vi "Save Project.vi"(0 "Project reference":refnum<vi>, 5 "MeasurementCore reference":refnum<vi>, 7 "Project path":path, 11 "error in (no error)":errorcluster) -> (15 "error out":errorcluster)   [LabVIEW 2021, in "Multiple Converter.lvlib"]
uses:
  Multiple Converter.lvlib
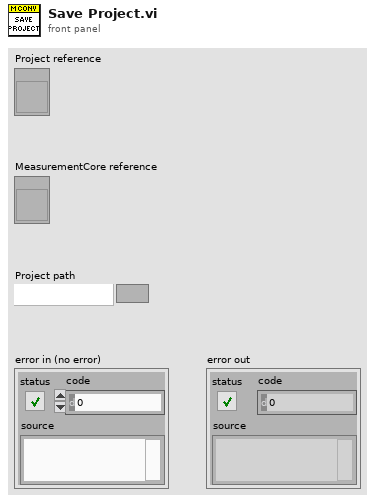
[diagram p1: front panel]
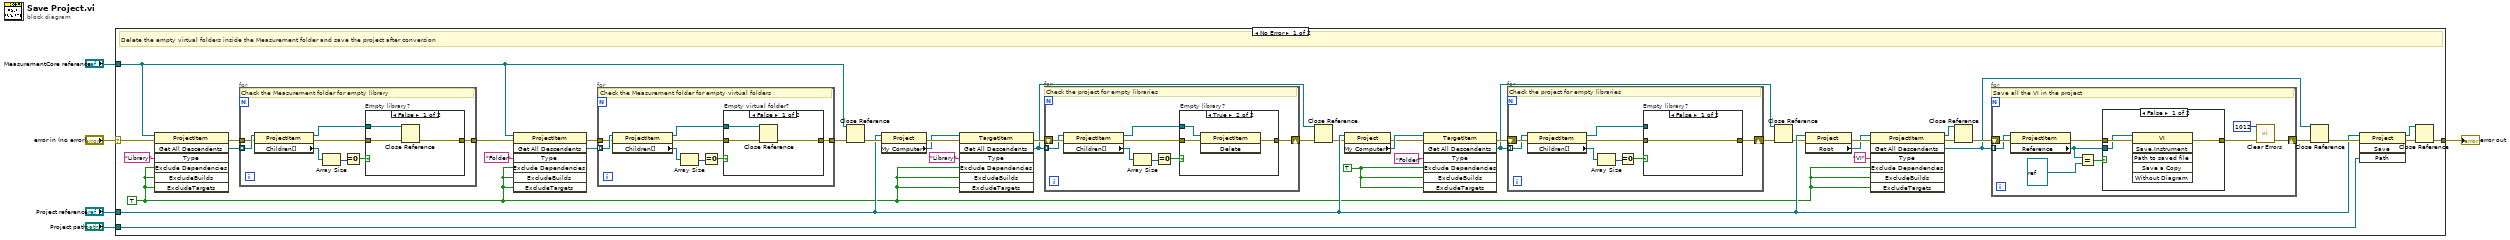
[diagram p0: block diagram]
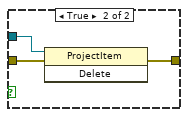
[diagram p2: hidden frame]
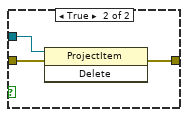
[diagram p3: hidden frame]
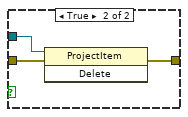
[diagram p4: hidden frame]
diagram:
  n1 = case shown="No Error" "error in (no error)" {
    selector: "error in (no error)" -> [w9 w112]
    tunnel: [w45 w112] -> w5
    tunnel: "Project path" -> [w41 _]
    tunnel: "MeasurementCore reference" -> [w6 _]
    tunnel: "Project reference" -> [w19 _]
    frame No Error {
      w7 = TRUE
      w18 = TRUE
      # "Delete the empty virtual folders inside the Measurement folder and save the project after conversion"
      n2 = invoke class="ProjectItem" method="Get All Descendents"(reference=w6, error in=w9, "Type"="Library", "Exclude Dependencies"=w7, "ExcludeBuilds"=w7, "ExcludeTargets"=w7) -> (error out=w11:errorcluster, "All Descendents"=w12:refnum<vi>[])  [unwired: 1 in, 5 out]
      n3 = for {
        tunnel: w12 -> [w54] mode=indexing
        tunnel: w11 -> [w53]
        tunnel: [w47] -> w8
        # "Check the Measurement folder for empty library"
        n4 = property class="ProjectItem"(reference=w54, error in=w53) -> (reference out=w48:refnum<vi>, error out=w50:errorcluster, "Children[]"=w52:refnum<vi>[])
        n5 = Array Size(array=w52) -> (size(s)=w51:i32)
        n6 = Equal To 0?(x=w51) -> (x = 0?=w49:bool)
        n7 = case "Empty library?" shown="False" w49 {
          tunnel: w50 -> [w57 w60]
          tunnel: w48 -> [w56 w59]
          tunnel: [w55 w58] -> w47
          frame False {
            n8 = Close Reference(reference=w56, error in (no error)=w57) -> (error out=w55:errorcluster)
          }
          frame True {
            n9 = invoke class="ProjectItem" method="Delete"(reference=w59, error in=w60) -> (error out=w58:errorcluster)  [unwired: 1 in, 2 out]
          }
        }
      }
      n10 = invoke class="ProjectItem" method="Get All Descendents"(reference=w6, error in=w8, "Type"="Folder", "Exclude Dependencies"=w7, "ExcludeBuilds"=w7, "ExcludeTargets"=w7) -> (error out=w42:errorcluster, "All Descendents"=w31:refnum<vi>[])  [unwired: 1 in, 5 out]
      n11 = for {
        tunnel: w31 -> [w80] mode=indexing
        tunnel: w42 -> [w79]
        tunnel: [w73] -> w24
        # "Check the Measurement folder for empty virtual folders"
        n12 = property class="ProjectItem"(reference=w80, error in=w79) -> (reference out=w74:refnum<vi>, error out=w76:errorcluster, "Children[]"=w78:refnum<vi>[])
        n13 = Array Size(array=w78) -> (size(s)=w77:i32)
        n14 = Equal To 0?(x=w77) -> (x = 0?=w75:bool)
        n15 = case "Empty virtual folder?" shown="False" w75 {
          tunnel: w76 -> [w83 w86]
          tunnel: w74 -> [w82 w85]
          tunnel: [w81 w84] -> w73
          frame False {
            n16 = Close Reference(reference=w82, error in (no error)=w83) -> (error out=w81:errorcluster)
          }
          frame True {
            n17 = invoke class="ProjectItem" method="Delete"(reference=w85, error in=w86) -> (error out=w84:errorcluster)  [unwired: 1 in, 2 out]
          }
        }
      }
      n18 = Close Reference(reference=w6, error in (no error)=w24) -> (error out=w23:errorcluster)
      n19 = property class="Project"(reference=w19, error in=w23) -> (error out=w35:errorcluster, "My Computer"=w25:refnum<vi>)  [unwired: 1 out]
      n20 = invoke class="TargetItem" method="Get All Descendents"(reference=w25, error in=w35, "Type"="Library", "Exclude Dependencies"=w7, "ExcludeBuilds"=w7, "ExcludeTargets"=w7) -> (error out=w33:errorcluster, "All Descendents"=w29:refnum<vi>[])  [unwired: 1 in, 5 out]
      n21 = for {
        shift-right: [w87] -> w30
        shift-left: w33 -> [w94]
        tunnel: w29 -> [w93] mode=indexing
        # "Check the project for empty libraries"
        n22 = property class="ProjectItem"(reference=w93, error in=w94) -> (reference out=w89:refnum<vi>, error out=w88:errorcluster, "Children[]"=w91:refnum<vi>[])
        n23 = Array Size(array=w91) -> (size(s)=w92:i32)
        n24 = Equal To 0?(x=w92) -> (x = 0?=w90:bool)
        n25 = case "Empty library?" shown="True" w90 {
          tunnel: w88 -> [w95 w98]
          tunnel: w89 -> [_ w97]
          tunnel: [w95 w96] -> w87
          frame False {
          }
          frame True {
            n26 = invoke class="ProjectItem" method="Delete"(reference=w97, error in=w98) -> (error out=w96:errorcluster)  [unwired: 1 in, 2 out]
          }
        }
      }
      n27 = Close Reference(reference=w29, error in (no error)=w30) -> (error out=w17:errorcluster)
      n28 = property class="Project"(reference=w19, error in=w17) -> (error out=w20:errorcluster, "My Computer"=w22:refnum<vi>)  [unwired: 1 out]
      n29 = invoke class="TargetItem" method="Get All Descendents"(reference=w22, error in=w20, "Type"="Folder", "Exclude Dependencies"=w18, "ExcludeBuilds"=w18, "ExcludeTargets"=w18) -> (error out=w16:errorcluster, "All Descendents"=w13:refnum<vi>[])  [unwired: 1 in, 5 out]
      n30 = for {
        shift-right: [w61] -> w15
        shift-left: w16 -> [w68]
        tunnel: w13 -> [w67] mode=indexing
        # "Check the project for empty libraries"
        n31 = property class="ProjectItem"(reference=w67, error in=w68) -> (reference out=w63:refnum<vi>, error out=w62:errorcluster, "Children[]"=w65:refnum<vi>[])
        n32 = Array Size(array=w65) -> (size(s)=w66:i32)
        n33 = Equal To 0?(x=w66) -> (x = 0?=w64:bool)
        n34 = case "Empty library?" shown="False" w64 {
          tunnel: w62 -> [w69 w72]
          tunnel: w63 -> [_ w71]
          tunnel: [w69 w70] -> w61
          frame False {
          }
          frame True {
            n35 = invoke class="ProjectItem" method="Delete"(reference=w71, error in=w72) -> (error out=w70:errorcluster)  [unwired: 1 in, 2 out]
          }
        }
      }
      n36 = Close Reference(reference=w13, error in (no error)=w15) -> (error out=w14:errorcluster)
      n37 = property class="Project"(reference=w19, error in=w14) -> (error out=w40:errorcluster, "Root"=w39:refnum<vi>)  [unwired: 1 out]
      n38 = invoke class="ProjectItem" method="Get All Descendents"(reference=w39, error in=w40, "Type"="VI", "Exclude Dependencies"=w7, "ExcludeBuilds"=w7, "ExcludeTargets"=w7) -> (reference out=w37:refnum<vi>, error out=w38:errorcluster, "All Descendents"=w26:refnum<vi>[])  [unwired: 1 in, 4 out]
      n39 = Close Reference(reference=w37, error in (no error)=w38) -> (error out=w36:errorcluster)
      n40 = for {
        shift-right: [w100] -> w28
        shift-left: w36 -> [w106]
        tunnel: w26 -> [w104] mode=indexing
        # "Save all the VI in the project"
        n41 = property class="ProjectItem"(reference=w104, error in=w106) -> (error out=w105:errorcluster, "Reference"=w101:refnum<vi>)  [unwired: 1 out]
        n42 = Equal?(x=w101, y=refnum<vi> refnum) -> (x = y?=w102:bool)
        n43 = case shown="False" w102 {
          tunnel: [w108 w111] -> w107
          tunnel: w105 -> [w110 w111]
          tunnel: w101 -> [w109 _]
          frame False {
            n44 = invoke class="VI" method="Save.Instrument"(reference=w109, error in=w110) -> (error out=w108:errorcluster)  [unwired: 4 in, 5 out]
          }
          frame True {
          }
        }
        n45 = call <vilib>:"Clear Errors.vi"("error in (no error)"=w107, "specific error code to clear (0: all)"=1012) -> ("error out"=w100:errorcluster)  [unwired: 4 in, 1 out]
      }
      n46 = Close Reference(reference=w26, error in (no error)=w28) -> (error out=w27:errorcluster)
      n47 = invoke class="Project" method="Save"(reference=w19, error in=w27, "Path"=w41) -> (reference out=w46:refnum<vi>, error out=w44:errorcluster)  [unwired: 1 in, 2 out]
      n48 = Close Reference(reference=w46, error in (no error)=w44) -> (error out=w45:errorcluster)
    }
    frame Error {
    }
  }
  "error out" <- w5
